vi "AI Propulsion.vi"(8 "error in (no error)":errorcluster, 11 "All Queue":T1) -> ()   [LabVIEW 2022 SP3]
uses:
  Controls/All Queue Ref.ctl
  Controls/ALL Health.ctl
  <vilib>/Utility/error.llb/DialogType.ctl
  6D_Global.vi
  <vilib>/DAQmx/miscellaneous.llb/DAQmx Fill In Error Info.vi
  <vilib>/DAQmx/read.llb/DAQmx Read (Analog 1D Wfm NChan NSamp).vi
  <vilib>/DAQmx/configure/timing.llb/DAQmx Timing (Sample Clock).vi
  <vilib>/DAQmx/create/channels.llb/DAQmx Create Channel (AI-Voltage-Basic).vi
  <vilib>/DAQmx/create/scale.llb/DAQmx Create Scale (Map Ranges).vi
  <resource>/objmgr/daqmx.rc
  <vilib>/DAQmx/configure/trigger.llb/DAQmx Start Trigger (Time).vi
panel:
  out "error out":errorcluster
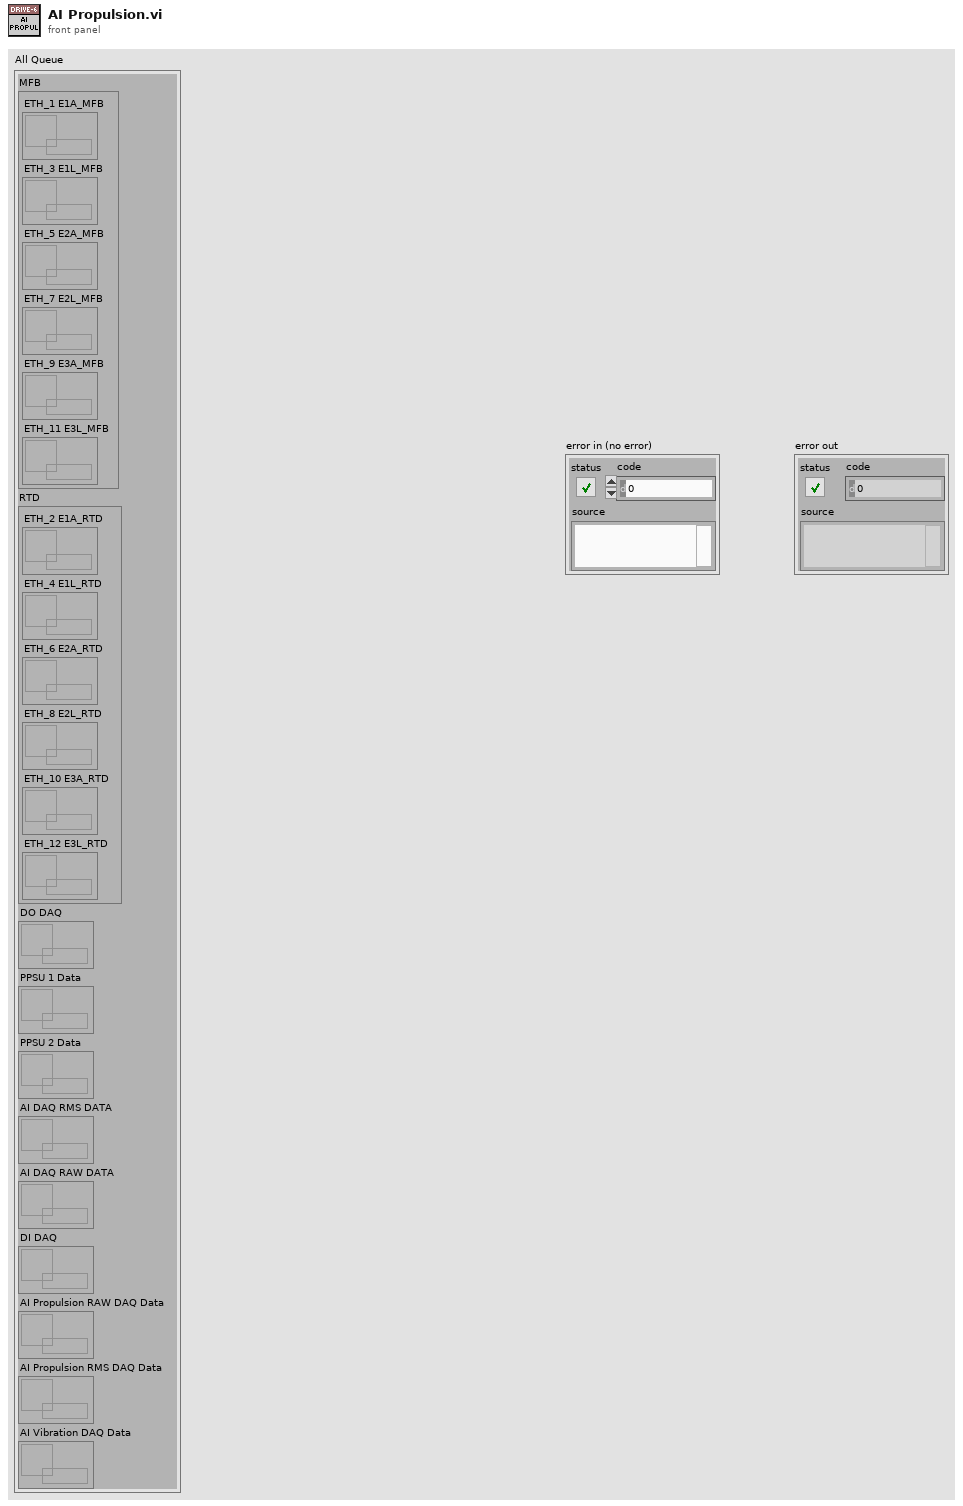
[diagram p1: front panel]
types:
  T1 = typedef "All Queue Ref.ctl" = cluster{"MFB":cluster{"ETH_1 E1A_MFB":refnum<queue>, "ETH_3 E1L_MFB":refnum<queue>, "ETH_5 E2A_MFB":refnum<queue>, "ETH_7 E2L_MFB":refnum<queue>, "ETH_9 E3A_MFB":refnum<queue>, "ETH_11 E3L_MFB":refnum<queue>}, "RTD":cluster{"ETH_2 E1A_RTD ":refnum<queue>, "ETH_4 E1L_RTD ":refnum<queue>, "ETH_6 E2A_RTD ":refnum<queue>, "ETH_8 E2L_RTD ":refnum<queue>, "ETH_10 E3A_RTD ":refnum<queue>, "ETH_12 E3L_RTD ":refnum<queue>}, "DO DAQ":refnum<queue>, "PPSU 1 Data":refnum<queue>, "PPSU 2 Data":refnum<queue>, "AI DAQ RMS DATA":refnum<queue>, "AI DAQ RAW DATA":refnum<queue>, "DI DAQ":refnum<queue>, "AI Propulsion RAW DAQ Data":refnum<queue>, "AI Propulsion RMS DAQ Data":refnum<queue>, "AI Vibration DAQ Data":refnum<queue>}
  T2 = enum16{"Channel Data Input", "Sampling Data Input", "Read Data", "Stop DAQ"}
  T3 = typedef "ALL Health.ctl" = enum16{"AI HS", "AI Vibration HS", "AI Propulsion HS", "DO HS", "Datalog HS", "PPSU HS", "ETH_1 DAQ", "ETH_1 RTD", "ETH_2 DAQ", "ETH_2 RTD", "ETH_5 RTD"}
  T4 = enum16{"Init", "Read 'All'", "Read 'n'", "Read '1'", "Write '1'", "Write 'n'", "Write 'All'"}
  T5 = cluster{"Samples per channel":i32, "Sampling Rate":dbl, "Sample Mode":i32, "Source":tag}
  T6 = cluster{"AI signal Lists":string, "AI Channel List":tag, "Prescale Min":dbl, "Prescale Max":dbl, "Sensor Min":dbl, "Sensor Max":dbl, "Units":string}[]
  T7 = typedef "DialogType.ctl" = u16
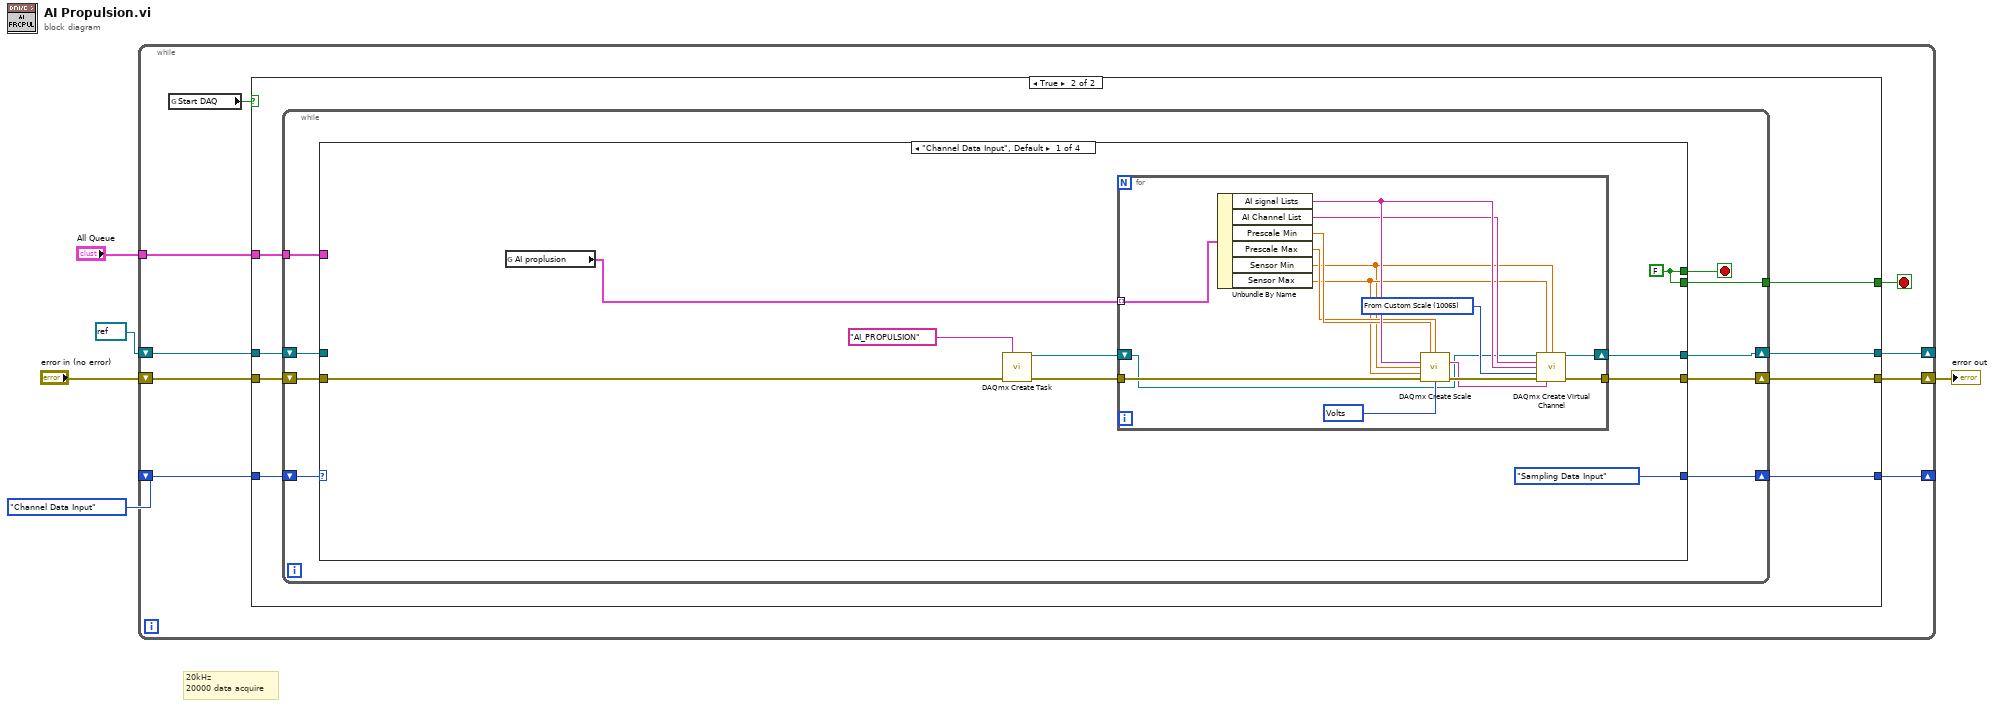
[diagram p0: block diagram]
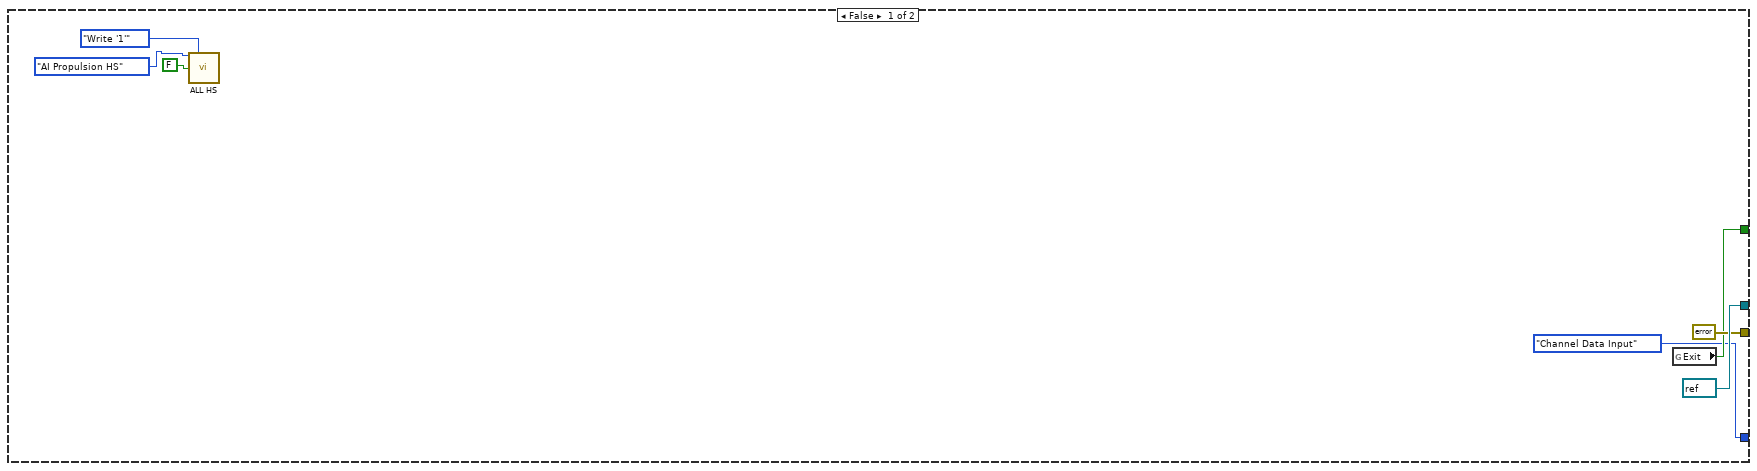
[diagram p2: hidden frame]
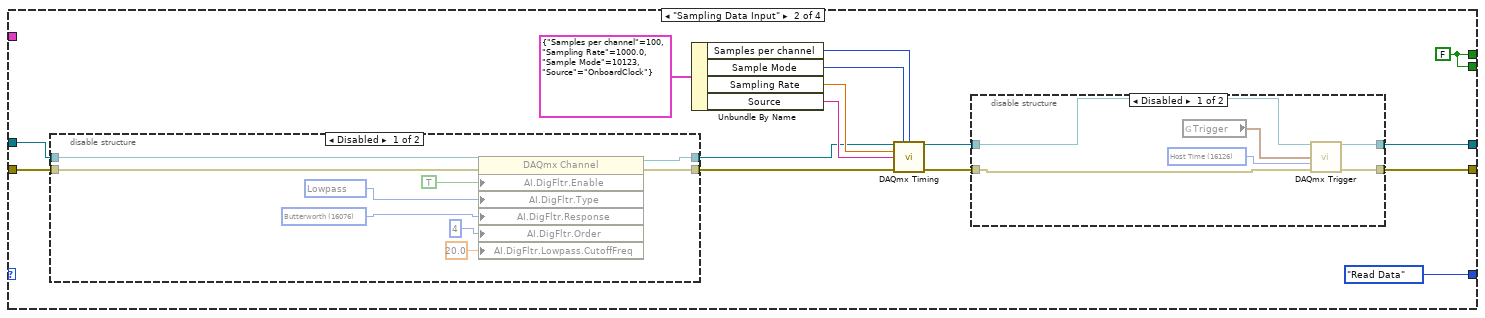
[diagram p3: hidden frame]
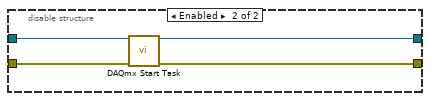
[diagram p5: hidden frame]
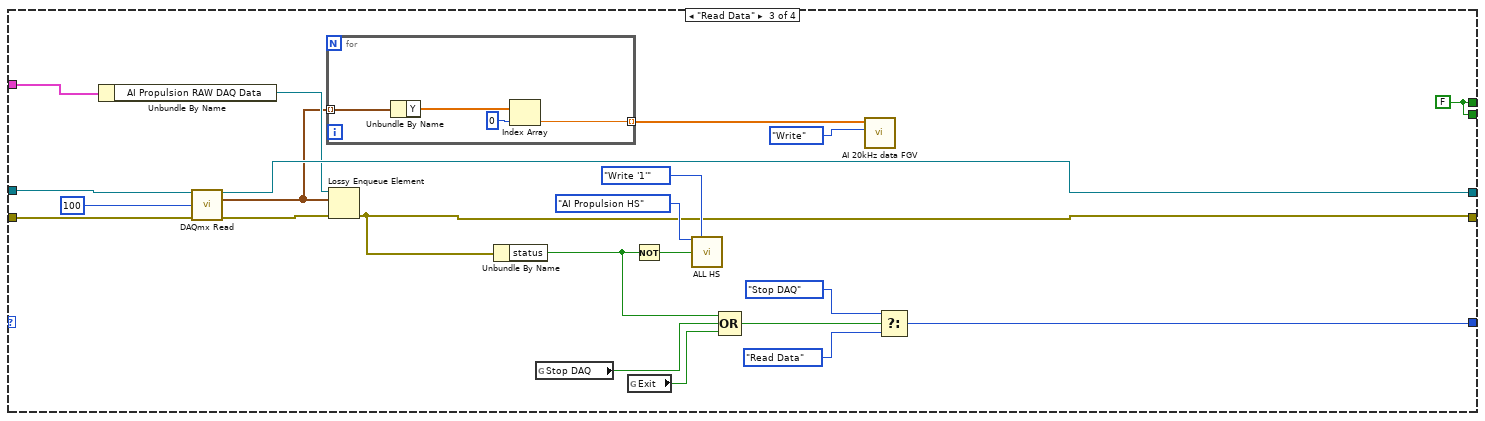
[diagram p6: hidden frame]
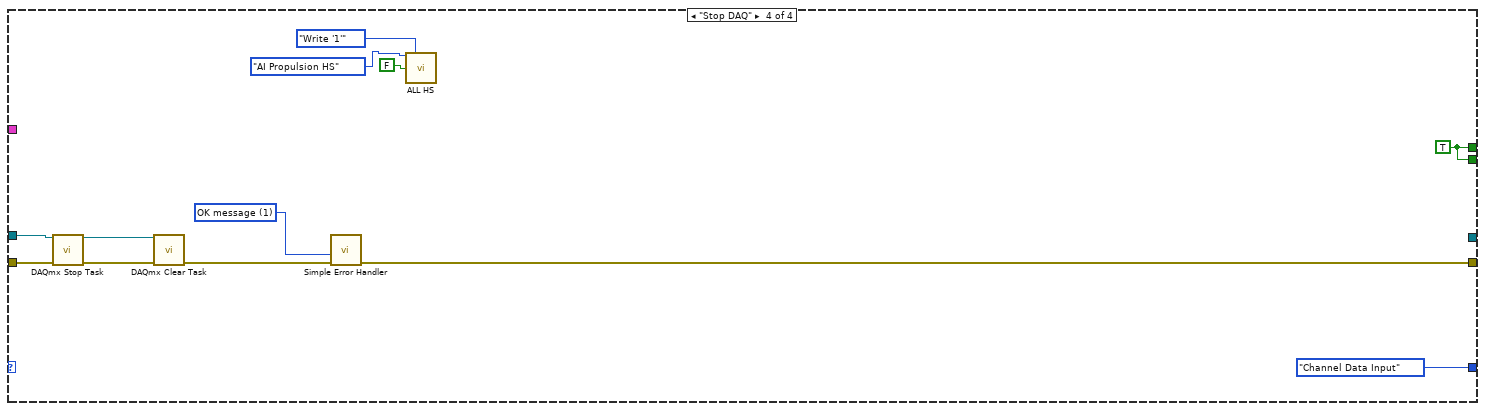
[diagram p7: hidden frame]
diagram:
  # "20kHz \n20000 data acquire"
  n1 = while {
    shift-right: [w11] -> _
    shift-left: T2."Channel Data Input" -> [w14]
    shift-right: [w13] -> _
    shift-left: refnum<k21> refnum ("task out") -> [w12]
    shift-right: [w8] -> w1
    shift-left: "error in (no error)" -> [w9]
    tunnel: "All Queue" -> [w7]
    stop <- w10 stop-if-true
    n2 = global read "6D_Global.vi" "Start DAQ"() -> (w6:bool)
    n3 = case shown="True" w6 {
      tunnel: w14 -> [_ w29]
      tunnel: [refnum<k21> refnum ("task out") w28] -> w13
      tunnel: w12 -> [_ w27]
      tunnel: [T2."Channel Data Input" w26] -> w11
      tunnel: [w19 w25] -> w10
      tunnel: w9 -> [_ w24]
      tunnel: [errorcluster {"status"=FALSE, "code"=0, "source"=""} ("error out") w22] -> w8
      tunnel: w7 -> [_ w23]
      frame False {
        n4 = call "ALL HS.vi"("Loop"=ALL_Health."AI Propulsion HS", "Option"=T4."Write '1'", "Status"=FALSE) -> ()  [unwired: 10 in, 3 out]
        n5 = global read "6D_Global.vi" "Exit"() -> (w19:bool)
      }
      frame True {
        n6 = while {
          tunnel: [w34] -> w25
          tunnel: w23 -> [w32]
          shift-right: [w35] -> w26
          shift-left: w29 -> [w38]
          shift-right: [w37] -> w28
          shift-left: w27 -> [w36]
          shift-right: [w31] -> w22
          shift-left: w24 -> [w33]
          stop <- w30 stop-if-true
          n7 = case shown="\"Channel Data Input\", Default" w38 {
            tunnel: w33 -> [w41 w67 w115 w136]
            tunnel: [w42 w71 w99 w128] -> w31
            tunnel: [w44 w72 w117 _] -> w37
            tunnel: w36 -> [_ w68 w116 w134]
            tunnel: [T2."Sampling Data Input" T2."Read Data" w118 T2."Channel Data Input"] -> w35
            tunnel: [w40 w63 w102 w125] -> w34
            tunnel: w32 -> [_ _ w107 _]
            tunnel: [w40 w63 w102 w125] -> w30
            frame "Channel Data Input", Default {
              w40 = FALSE
              n8 = global read "6D_Global.vi" "AI proplusion"() -> (w39:T6)
              n9 = call <vilib>:"DAQmx Create Task.vi"("new task name"="AI_PROPULSION", "error in"=w41) -> ("task out"=w47:refnum<k21>, "error out"=w46:errorcluster)  [unwired: 12 in]
              n10 = for {
                tunnel: w46 -> [w62]
                tunnel: w39 -> [w60] mode=indexing
                shift-right: [w50] -> w44
                shift-left: w47 -> [w49]
                tunnel: [w48] -> w42
                w51 = 10065 items=["Volts"=10348, "From Custom Scale"=10065] ("units")
                w52 = 10348 items=["Volts"=10348, "Amps"=10342, "Deg F"=10144, "Deg C"=10143, "Deg R"=10145, "Kelvins"=10325, "Strain"=10299, "Ohms"=10384, "Hz"=10373, "Seconds"=10364, "Meters"=10219, "Inches"=10379, "Degrees"=10146, "Radians"=10273, "Ticks"=10304, "g"=10186, "m/s^2"=12470, "m/s"=15959, "in/s"=15960, "Pascals"=10081, "Newtons"=15875, "Pounds"=15876, "kgf"=15877, "psi"=15879, "bar"=15880, "Nm"=15881, "oz-in"=15882, "lb-in"=15883, "lb-ft"=15884, "Volts/Volt"=15896, "mVolts/Volt"=15897, "pCoulombs"=16103, "Coulombs"=16102, "From TEDS"=12516] ("pre-scaled units")
                n11 = Unbundle By Name(w60) -> ("AI signal Lists"=w59:string, "AI Channel List"=w58:tag, "Prescale Min"=w56:dbl, "Prescale Max"=w55:dbl, "Sensor Min"=w53:dbl, "Sensor Max"=w54:dbl)
                n12 = call-poly <vilib>:"DAQmx Create Scale.vi"("pre-scaled minimum"=w56, "pre-scaled maximum"=w55, "name"=w59, "scaled minimum"=w53, "scaled maximum"=w54, "error in"=w62, "pre-scaled units"=w52) -> ("scale out"=w57:tag, "error out"=w61:errorcluster)  [unwired: 7 in]
                n13 = call-poly <vilib>:"DAQmx Create Virtual Channel.vi"("task in"=w49, "maximum value"=w54, "minimum value"=w53, "physical channels"=w58, "name to assign"=w59, "units"=w51, "error in"=w61, "custom scale name"=w57) -> ("task out"=w50:refnum<k21>, "error out"=w48:errorcluster)  [unwired: 6 in]
              }
            }
            frame "Sampling Data Input" {
              w63 = FALSE
              n14 = disable-structure shown="Disabled" {
                disable-tunnel: [w86 w88] -> w69
                disable-tunnel: w68 -> [w85 w88]
                disable-tunnel: w67 -> [w84 w87]
                disable-tunnel: [w83 w87] -> w66
                frame Disabled {
                  w80 = 16076 items=["Constant Group Delay"=16075, "Butterworth"=16076, "Elliptical"=16077, "Hardware Defined"=10191] ("AI.DigFltr.Response")
                  w81 = 16071 items=["Lowpass"=16071, "Highpass"=16072, "Bandpass"=16073, "Notch"=16074, "Custom"=10137] ("AI.DigFltr.Type")
                  n15 = property class="DAQmx Channel"(reference=w85, error in=w84, "AI.DigFltr.Enable"=TRUE ("AI.Lowpass.Enable"), "AI.DigFltr.Type"=w81, "AI.DigFltr.Response"=w80, "AI.DigFltr.Order"=u32 4, "AI.DigFltr.Lowpass.CutoffFreq"=20.0) -> (reference out=w86:refnum<k21>, error out=w83:errorcluster)
                }
                frame Enabled {
                }
              }
              n16 = Unbundle By Name(T5 {"Samples per channel"=100, "Sampling Rate"=1000.0, "Sample Mode"=10123, "Source"="OnboardClock"} ("Analog Input Samples Data")) -> ("Samples per channel"=w74:i32, "Sample Mode"=w75:i32, "Sampling Rate"=w76:dbl, "Source"=w77:tag)
              n17 = call-poly <vilib>:"DAQmx Timing.vi"("task/channels in"=w69, "sample mode"=w75, "samples per channel"=w74, "rate"=w76, "source"=w77, "error in"=w66) -> ("task out"=w65:refnum<k21>, "error out"=w64:errorcluster)  [unwired: 8 in]
              n18 = disable-structure shown="Disabled" {
                disable-tunnel: w65 -> [w94 w97]
                disable-tunnel: w64 -> [w93 w98]
                disable-tunnel: [w92 w96] -> w72
                disable-tunnel: [w91 w95] -> w71
                frame Disabled {
                  w90 = 16126 items=["Host Time"=16126, "I/O Device Time"=16127] ("timescale")
                  n19 = global read "6D_Global.vi" "Trigger"() -> (w89:timestamp)
                  n20 = call-poly <vilib>:"DAQmx Trigger.vi"("task/channels in"=w94, "when"=w89, "timescale"=w90, "error in"=w93) -> ("task out"=w92:refnum<k21>, "error out"=w91:errorcluster)  [unwired: 10 in]
                }
                frame Enabled {
                  n21 = call <vilib>:"DAQmx Start Task.vi"("task/channels in"=w97, "error in"=w98) -> ("task out"=w96:refnum<k21>, "error out"=w95:errorcluster)  [unwired: 12 in]
                }
              }
            }
            frame "Read Data" {
              w102 = FALSE
              n22 = Unbundle By Name(w107) -> ("AI Propulsion RAW DAQ Data"=w104:refnum<queue>)
              n23 = call-poly <vilib>:"DAQmx Read.vi"("task/channels in"=w116, "number of samples per channel"=100, "error in"=w115) -> ("task out"=w117:refnum<k21>, "data"=w101:waveform(dbl)[], "error out"=w100:errorcluster)  [unwired: 10 in]
              n24 = for {
                tunnel: w101 -> [w122] mode=indexing
                tunnel: [w121] -> w105 mode=indexing
                n25 = Unbundle By Name(w122) -> ("Y"=w123:dbl[])
                n26 = Index Array(array=w123, index=0) -> (element=w121:dbl)
              }
              n27 = Lossy Enqueue Element(queue=w104, element=w101, error in (no error)=w100) -> (error out=w99:errorcluster)  [unwired: 3 out]
              n28 = Unbundle By Name(w99) -> ("status"=w109:bool)
              n29 = global read "6D_Global.vi" "Stop DAQ"() -> (w112:bool)
              n30 = global read "6D_Global.vi" "Exit"() -> (w113:bool)
              n31 = Not(x=w109) -> (.not. x?=w110:bool)
              n32 = call "ALL HS.vi"("Loop"=ALL_Health."AI Propulsion HS", "Option"=T4."Write '1'", "Status"=w110) -> ()  [unwired: 10 in, 3 out]
              n33 = Compound Arithmetic op=OR(w109, w112, w113) -> (w108:bool)
              n34 = call "AI 20kHz data FGV.vi"("Enum"=enum16{"Read", "Write"}."Write", "Propulsion Data"=w105) -> ()  [unwired: 8 in, 2 out]
              n35 = Select(t=T2."Stop DAQ", s=w108, f=T2."Read Data") -> (s? t:f=w118:T2)
            }
            frame "Stop DAQ" {
              w125 = TRUE
              w132 = T7 1 items=["no dialog", "OK message", "continue or stop message", "OK message + warnings", "continue/stop + warnings"] ("type of dialog (OK msg:1)")
              n36 = call <vilib>:"DAQmx Stop Task.vi"("task/channels in"=w134, "error in"=w136) -> ("task out"=w133:refnum<k21>, "error out"=w135:errorcluster)  [unwired: 12 in]
              n37 = call <vilib>:"DAQmx Clear Task.vi"("task in"=w133, "error in"=w135) -> ("error out"=w131:errorcluster)  [unwired: 13 in]
              n38 = call <vilib>:"Simple Error Handler.vi"("type of dialog (OK msg:1)"=w132, "error in (no error)"=w131) -> ("error out"=w128:errorcluster)  [unwired: 3 in, 4 out]
              n39 = call "ALL HS.vi"("Loop"=ALL_Health."AI Propulsion HS", "Option"=T4."Write '1'", "Status"=FALSE) -> ()  [unwired: 10 in, 3 out]
            }
          }
        }
      }
    }
  }
  "error out" <- w1
